vi "Read Manager.vi"(8 "error in (no error)":errorcluster, 10 "Protocol Queue":refnum<class "Message Enqueuer.lvclass">, 11 "MFC in":refnum<class "MFC.lvclass">) -> (0 "error out":errorcluster, 3 "MFC out":refnum<class "MFC.lvclass">)   [LabVIEW 2013]
uses:
  MFC.lvclass
  MFC Messages/Write Protocol Msg/Write Protocol Msg.lvclass
  <vilib>/ActorFramework/Actor/Actor.lvclass
  <vilib>/ActorFramework/Message Enqueuer/Message Enqueuer.lvclass
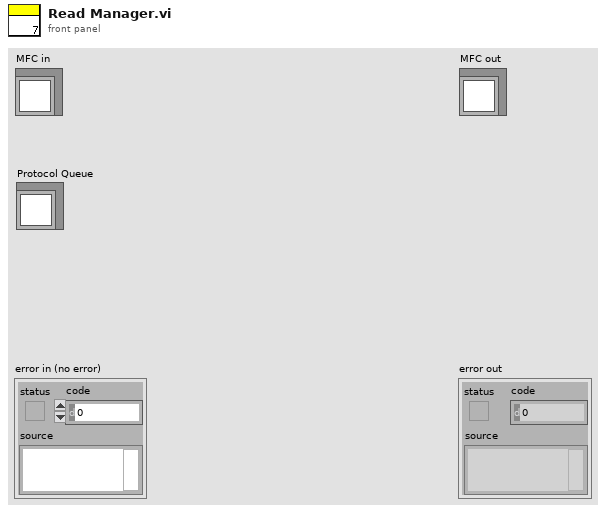
[diagram p1: front panel]
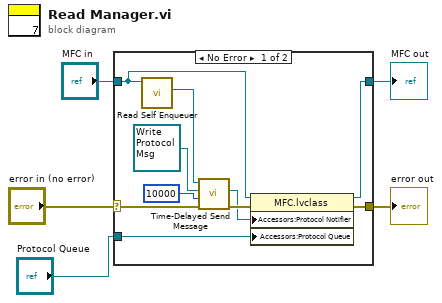
[diagram p0: block diagram]
diagram:
  n1 = case shown="No Error" "error in (no error)" {
    selector: "error in (no error)" -> [w11 w17]
    tunnel: [w13 w17] -> w2
    tunnel: [w14 w16] -> w3
    tunnel: "MFC in" -> [w7 w16]
    tunnel: "Protocol Queue" -> [w9 _]
    frame No Error {
      n2 = call <vilib>:"Read Self Enqueuer.vi"("Actor"=w7) -> ("Self Enqueuer"=w6:refnum<class "Message Enqueuer.lvclass">)  [unwired: 10 in]
      n3 = call <vilib>:"Time-Delayed Send Message.vi"("error in (no error)"=w11, "Milliseconds To Wait"=10000, "Message"=refnum<class "Write Protocol Msg.lvclass"> refnum ("MFC Actor.lvlib:Write Protocol Msg.lvclass"), "Message Enqueuer"=w6) -> ("error out"=w12:errorcluster, "Delivery Notifier"=w10:refnum<notifier>)  [unwired: 6 in]
      n4 = property class="MFC.lvclass"(reference=w7, error in=w12, "Accessors:Protocol Notifier"=w10, "Accessors:Protocol Queue"=w9) -> (reference out=w14:refnum<class "MFC.lvclass">, error out=w13:errorcluster)
    }
    frame Error {
    }
  }
  "error out" <- w2
  "MFC out" <- w3
